vi "count time to cycles.vi"(4 "dispmsg?":bool=TRUE caption="Display Message (T)", 6 "Trigger Freq":dbl[unit]=42077.399999999994, 7 "Count Time Set":dbl[unit]=1.0 min=0.0 max=10000.0 step=1.0 format="%#_7g") -> (0 "changed?":bool, 2 "Count Time Current":dbl[unit]=1.0 min=0.0 max=10000.0 step=1.0 format="%#_7g", 3 "Number of triggers":dbl caption="Cycles")   [LabVIEW 2015]
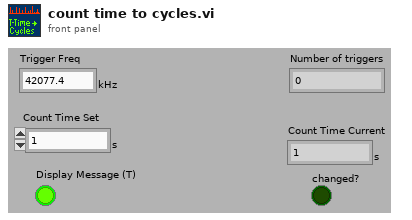
[diagram p1: front panel]
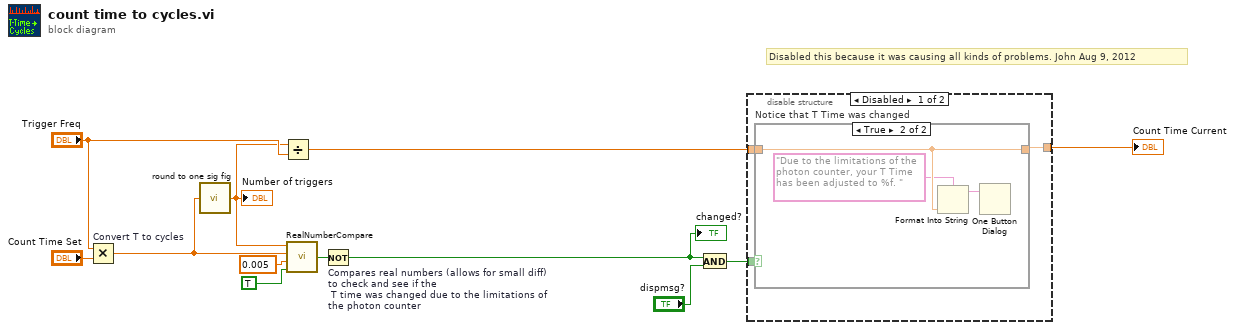
[diagram p0: block diagram]
diagram:
  # "Disabled this because it was causing all kinds of problems. John Aug 9, 2012"
  n1 = Multiply "Convert T to cycles"(x="Trigger Freq", y="Count Time Set") -> (x*y=w3:dbl)
  n2 = call "round to one sig fig.vi"("input number"=w3) -> ("rounded to 1 sig fig"=w1:dbl)
  "Number of triggers" <- w1
  n3 = Divide(x=w1, y="Trigger Freq") -> (x/y=w2:dbl[unit])
  n4 = call "RealNumberCompare.vi"("Percent? (Default F)"=TRUE, "Difference?"=0.005, "Number 2"=w3, "Number 1"=w1) -> ("Equal to?"=w9:bool)
  n5 = Not "Compares real numbers (allows for small diff) to check and see if the\n T time was changed due to the limitations of the photon counter"(x=w9) -> (.not. x?=w5:bool)
  "changed?" <- w5
  n6 = And(x=w5, y="dispmsg?") -> (x .and. y?=w7:bool)
  n7 = disable-structure shown="Disabled" {
    disable-tunnel: w7 -> [w15 _]
    disable-tunnel: [w14 w20] -> w6
    disable-tunnel: w2 -> [w13 w20]
    frame Disabled {
      n8 = case "Notice that T Time was changed" shown="True" w15 {
        tunnel: w13 -> [w16 w19]
        tunnel: [w16 w19] -> w14
        frame False {
        }
        frame True {
          n9 = Format Into String(format string="Due to the limitations of the photon counter, your T Time has been adjusted to %f. ", w19) -> (resulting string=w17:string)  [unwired: 2 in, 1 out]
          n10 = One Button Dialog(message=w17) -> ()  [unwired: 2 out]
        }
      }
    }
    frame Enabled {
    }
  }
  "Count Time Current" <- w6
